vi "IND560 Read Unstable Weight.vi"(8 "Error In":errorcluster, 11 "read buffer":string) -> (0 "Error Out":errorcluster, 1 "IND560 Selector":T1, 2 "Displayed Gross Wt.":dbl=2.91, 3 "Displayed Net Wt.":dbl=0.04)   [LabVIEW 2020]
uses:
  Type Definitions/IND560 Data Output Selector.ctl
panel:
  out "wt0102 (Displayed Net Wt.)":dbl[](array[numeric])
  out "wt0101 (Displayed Gross Wt.)":dbl[](array[numeric])
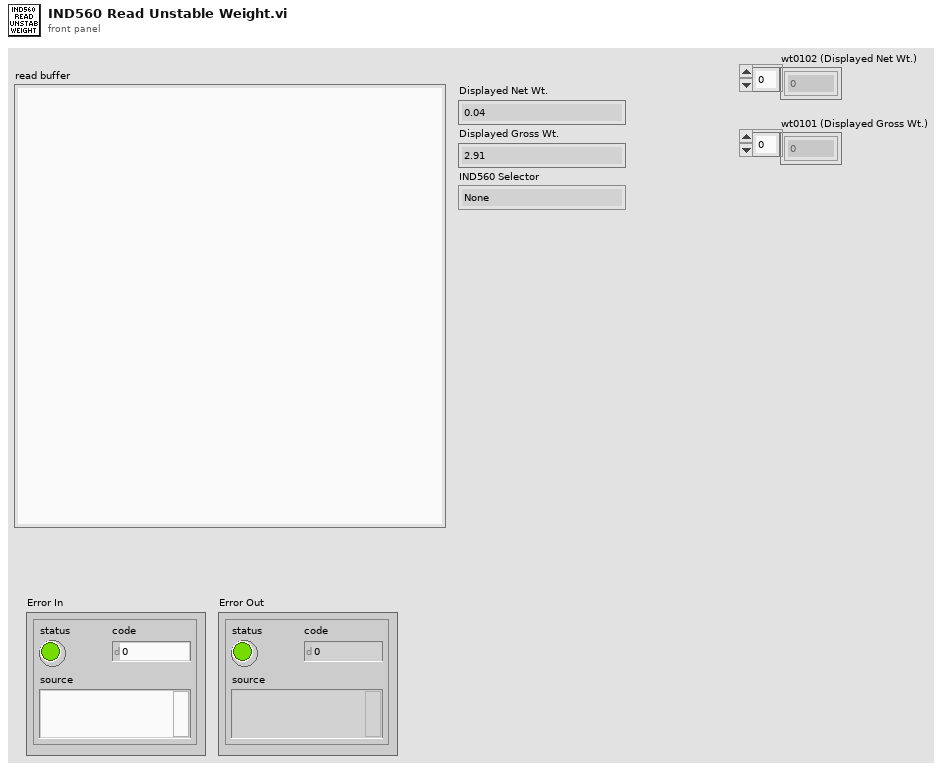
[diagram p1: front panel]
types:
  T1 = typedef "IND560 Data Output Selector.ctl" = enum16{"None", "Use Gross Not Equal Net", "Use Gross Equal Net", "Use Unstable Weights"}
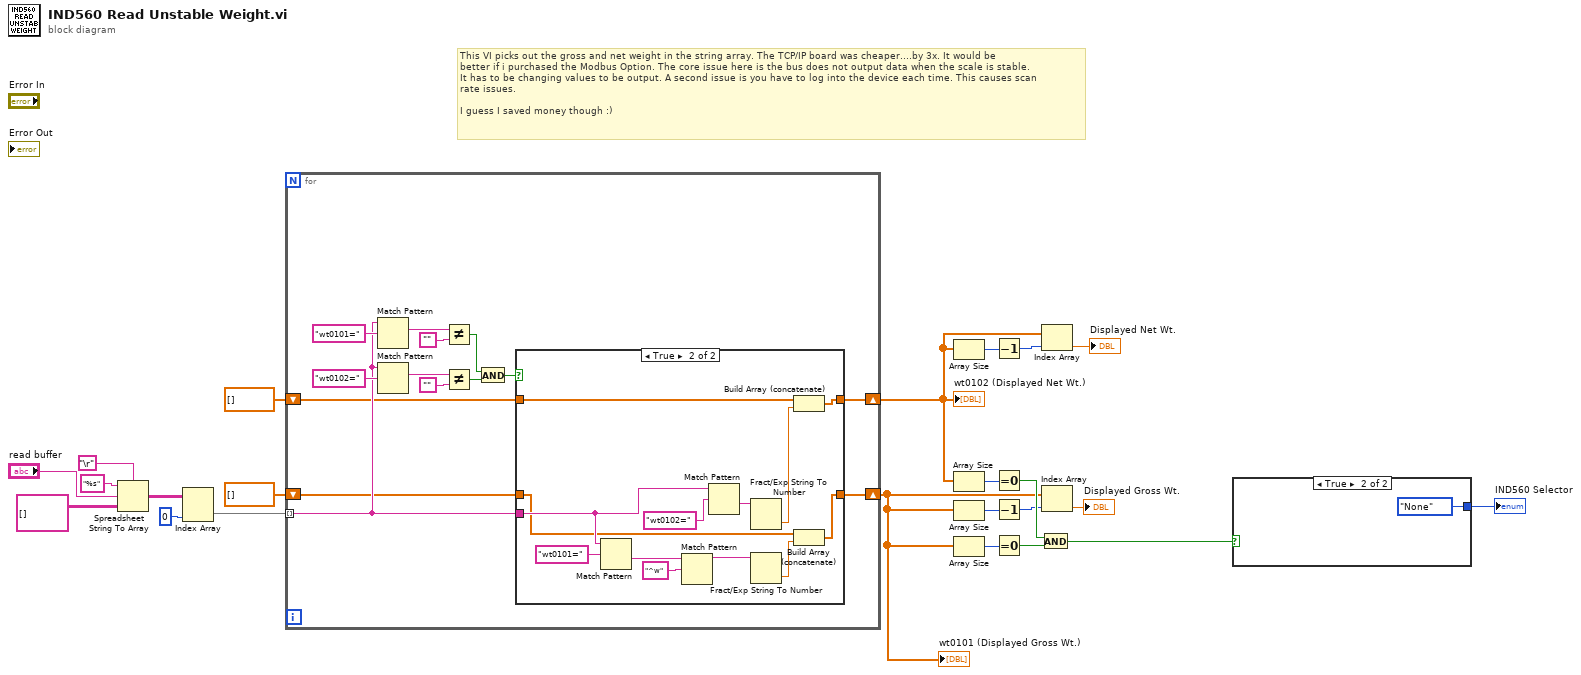
[diagram p0: block diagram]
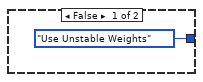
[diagram p2: hidden frame]
diagram:
  # "This VI picks out the gross and net weight in the string array. The TCP/IP board was cheaper....by 3x. It would be\nbetter if i purchased the Modbus Option. The core issue here is the bus does not output data when the scale is stable.\nIt has to be changing values to be output. A second issue is you have to log into the device each time. This causes scan\nrate issues.\n\nI guess I saved money though :)"
  n1 = Spreadsheet String To Array(delimiter (Tab)="\r", format string="%s", spreadsheet string="read buffer", array type (2D Dbl)=string[][] []) -> (array=w22:string[][])
  n2 = Index Array(array=w22, index (col)=0 ("disabled index (col)")) -> (element=w16:string[])  [unwired: 1 in]
  n3 = for {
    tunnel: w16 -> [w28] mode=indexing
    shift-right: [w26] -> w5
    shift-left: dbl[] [] -> [w27]
    shift-right: [w24] -> w6
    shift-left: dbl[] [] -> [w25]
    n4 = Match Pattern(string=w28, regular expression="wt0101=") -> (match substring=w34:string)  [unwired: 1 in, 3 out]
    n5 = Match Pattern(string=w28, regular expression="wt0102=") -> (match substring=w35:string)  [unwired: 1 in, 3 out]
    n6 = Not Equal?(x=w34, y="") -> (x != y?=w31:bool)
    n7 = Not Equal?(x=w35, y="") -> (x != y?=w30:bool)
    n8 = And(x=w31, y=w30) -> (x .and. y?=w29:bool)
    n9 = case shown="True" w29 {
      tunnel: w28 -> [_ w47]
      tunnel: w27 -> [w39 w45]
      tunnel: [w39 w44] -> w26
      tunnel: w25 -> [w38 w42]
      tunnel: [w38 w41] -> w24
      frame False {
      }
      frame True {
        n10 = Match Pattern(string=w47, regular expression="wt0101=") -> (after substring=w51:string)  [unwired: 1 in, 3 out]
        n11 = Match Pattern(string=w51, regular expression="^w") -> (before substring=w49:string)  [unwired: 1 in, 3 out]
        n12 = Match Pattern(string=w47, regular expression="wt0102=") -> (after substring=w46:string)  [unwired: 1 in, 3 out]
        n13 = Fract/Exp String To Number(string=w46) -> (number=w40:dbl)  [unwired: 3 in, 1 out]
        n14 = Fract/Exp String To Number(string=w49) -> (number=w43:dbl)  [unwired: 3 in, 1 out]
        n15 = Build Array (concatenate)(w42, w40) -> (w41:dbl[])
        n16 = Build Array (concatenate)(w45, w43) -> (w44:dbl[])
      }
    }
  }
  "wt0101 (Displayed Gross Wt.)" <- w5
  "wt0102 (Displayed Net Wt.)" <- w6
  n17 = Array Size(array=w6) -> (size(s)=w9:i32)
  n18 = Array Size(array=w6) -> (size(s)=w11:i32)
  n19 = Array Size(array=w5) -> (size(s)=w7:i32)
  n20 = Array Size(array=w5) -> (size(s)=w12:i32)
  n21 = Decrement(x=w9) -> (x-1=w10:i32)
  n22 = Equal To 0?(x=w11) -> (x = 0?=w13:bool)
  n23 = Decrement(x=w7) -> (x-1=w8:i32)
  n24 = Equal To 0?(x=w12) -> (x = 0?=w14:bool)
  n25 = And(x=w13, y=w14) -> (x .and. y?=w4:bool)
  n26 = Index Array(array=w6, index=w10) -> (element=→"Displayed Net Wt.":dbl)
  n27 = Index Array(array=w5, index=w8) -> (element=→"Displayed Gross Wt.":dbl)
  n28 = case shown="True" w4 {
    tunnel: [IND560_Data_Output_Selector."Use Unstable Weights" ("IND560 Selector") IND560_Data_Output_Selector."None" ("IND560 Selector")] -> w1
    frame False {
    }
    frame True {
    }
  }
  "IND560 Selector" <- w1
